vi "Set Parent Window.vi"(8 "error in (no error)":errorcluster, 10 "new parent":u32, 11 "child":u32) -> (0 "error out":errorcluster)   [LabVIEW 2009]
uses:
  USER32.DLL
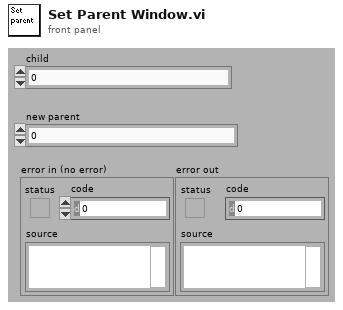
[diagram p1: front panel]
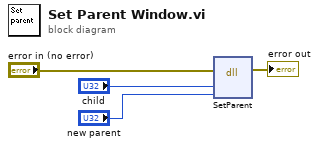
[diagram p0: block diagram]
diagram:
  n1 = dll-call lib="user32.dll" fn="SetParent"(error in="error in (no error)", "Child"="child", "NewParent"="new parent") -> (error out=→"error out":errorcluster)  [unwired: 4 in, 2 out]
